vi "format_string2arcmin.vi"(7 "Arcmin-Str":string) -> (8 "Arcmin":dbl format="%.2g")   [LabVIEW 2011]
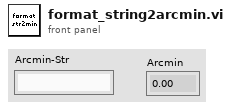
[diagram p1: front panel]
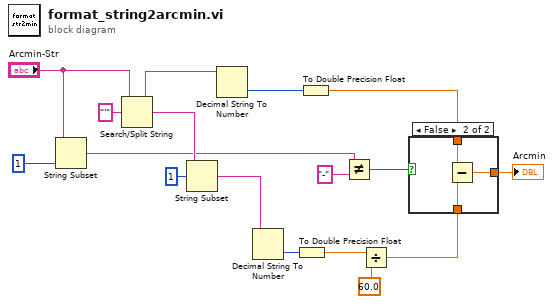
[diagram p0: block diagram]
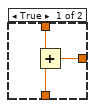
[diagram p2: hidden frame]
diagram:
  n1 = String Subset(string="Arcmin-Str", length (rest)=1 ("offset (0)")) -> (substring=w3:string)  [unwired: 1 in]
  n2 = Search/Split String(string="Arcmin-Str", search string/char (-)="'") -> (substring before match=w14:string, match + rest of string=w16:string)  [unwired: 1 in, 1 out]
  n3 = String Subset(string=w16, offset (0)=1) -> (substring=w13:string)  [unwired: 1 in]
  n4 = Decimal String To Number(string=w14) -> (number=w5:i32)  [unwired: 2 in, 1 out]
  n5 = Decimal String To Number(string=w13) -> (number=w12:i32)  [unwired: 2 in, 1 out]
  n6 = To Double Precision Float(number=w12) -> (double precision float=w11:dbl)
  n7 = To Double Precision Float(number=w5) -> (double precision float=w9:dbl)
  n8 = Not Equal?(x=w3, y="-") -> (x != y?=w6:bool)
  n9 = Divide(x=w11, y=60.0) -> (x/y=w8:dbl)
  n10 = case shown="False" w6 {
    tunnel: w9 -> [w20 w23]
    tunnel: w8 -> [w19 w22]
    tunnel: [w18 w21] -> w7
    frame True {
      n11 = Add(x=w20, y=w19) -> (x+y=w18:dbl)
    }
    frame False {
      n12 = Subtract(x=w23, y=w22) -> (x-y=w21:dbl)
    }
  }
  "Arcmin" <- w7
